vi "Update UI List.vi"(8 "error in (no error)":errorcluster, 11 "Data Cluster":T1 {"Pump_data"."mix rpm" format="%.2f"; "Pump_data"."Volume corrected" format="%.2f"; "Pump_data"."Position_MM" format="%.3f"; "Pump_data"."Volume PV" format="%.2f"; "Pump_data"."Flow PV" format="%#.6f"; "Pump_data"."Pressure PV" format="%.3f"}) -> (0 "error out":errorcluster, 3 "Data Cluster 2":T1 {"Pump_data"."mix rpm" format="%.2f"; "Pump_data"."Volume corrected" format="%.2f"; "Pump_data"."Position_MM" format="%.3f"; "Pump_data"."Volume PV" format="%.2f"; "Pump_data"."Flow PV" format="%#.6f"; "Pump_data"."Pressure PV" format="%.3f"})   [LabVIEW 2023, in "AutoPV.lvlib"]
uses:
  AutoPV.lvlib
  Module Data--cluster.ctl
  <vilib>/ActorFramework/Message Enqueuer/Message Enqueuer.lvclass
  Drive/Pump_Data_Type.ctl
  Initial Data/InitalData Type.ctl
  Drive/Drive.lvlib
  Initial Data/Initial Data.lvlib
panel:
  # "Образец"
  # "Образец"
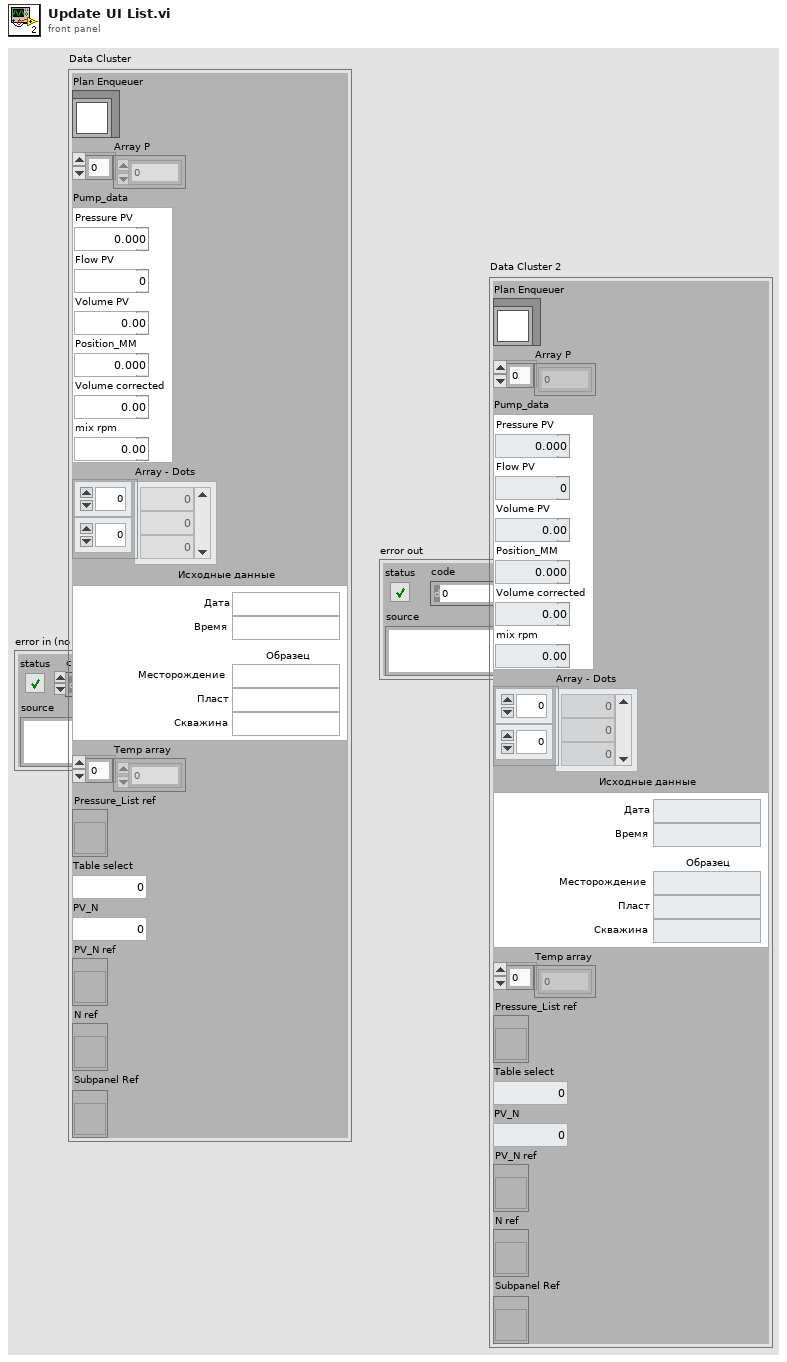
[diagram p1: front panel]
types:
  T1 = typedef "AutoPV.lvlib/Module Data--cluster.ctl" = cluster{"Plan Enqueuer":refnum<class "Message Enqueuer.lvclass">, "Array P":dbl[], "Pump_data":T2, "Array - Dots":dbl[][], "Исходные данные":T3, "Temp array":dbl[], "Pressure_List ref":refnum<vi>, "Table select":i32, "PV_N":i32, "PV_N ref":refnum<vi>, "N ref":refnum<vi>, "Subpanel Ref":refnum<vi>}
  T2 = typedef "Drive.lvlib/Pump_Data_Type.ctl" = cluster{"Pressure PV":dbl, "Flow PV":dbl, "Volume PV":dbl, "Position_MM":dbl, "Volume corrected":dbl, "mix rpm":dbl}
  T3 = typedef "Initial Data.lvlib/InitalData Type.ctl" = cluster{"Дата":string, "Время":string, "Месторождение":string, "Пласт":string, "Скважина":string}
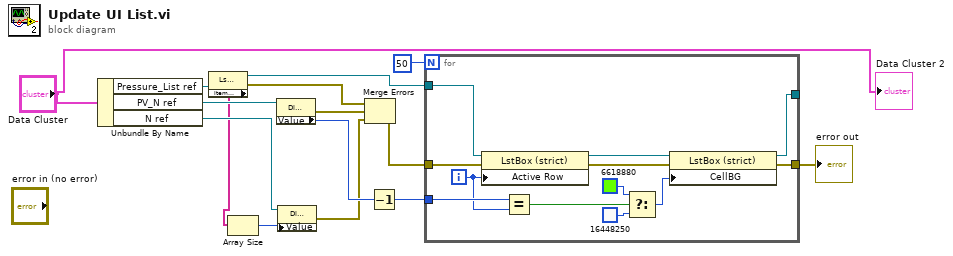
[diagram p0: block diagram]
diagram:
  n1 = Unbundle By Name("Data Cluster") -> ("Pressure_List ref"=w7:refnum<vi>, "PV_N ref"=w13:refnum<vi>, "N ref"=w8:refnum<vi>)
  n2 = property class="LstBox (strict)"(reference=w7) -> (reference out=w4:refnum<vi>, error out=w5:errorcluster, "Item Names"=w1:string[])  [unwired: 1 in]
  n3 = Array Size(array=w1) -> (size(s)=w2:i32)
  n4 = property class="DigNum (strict)"(reference=w13) -> (error out=w12:errorcluster, "Value"=w11:u32)  [unwired: 1 in, 1 out]
  n5 = property class="DigNum (strict)"(reference=w8, "Value"=w2) -> (error out=w3:errorcluster)  [unwired: 1 in, 1 out]
  n6 = Merge Errors(w5, w12, w3) -> (w6:errorcluster)
  n7 = Decrement(x=w11) -> (x-1=w10:u32)
  n8 = for {
    N: 50 -> [_]
    tunnel: w6 -> [w27]
    tunnel: w4 -> [w26]
    tunnel: [w25] -> _
    tunnel: [w24] -> w14
    tunnel: w10 -> [w23]
    i -> [w16]
    n9 = property class="LstBox (strict)"(reference=w26, error in=w27, "Active Row"=w16) -> (reference out=w22:refnum<vi>, error out=w21:errorcluster)
    n10 = Equal?(x=w23, y=w16) -> (x = y?=w17:bool)
    n11 = Select(t=u32 6618880, s=w17, f=u32 16448250) -> (s? t:f=w18:u32)
    n12 = property class="LstBox (strict)"(reference=w22, error in=w21, "CellBG"=w18) -> (reference out=w25:refnum<vi>, error out=w24:errorcluster)
  }
  "error out" <- w14
  "Data Cluster 2" <- "Data Cluster"
